vi "Save File Product Header Specific.vi"(8 "Error In":errorcluster, 10 "LV Program":T7=enum."DOE Stand", 11 "Appliance Details":T1 {"Dryer"."Dryer Initial IMC Data"."Maximum Weight (lbf)" format="%03_6g"; "Dryer"."Dryer Initial IMC Data"."Average Weight (lbf)" format="%03_6g"; "Dryer"."Dryer Initial IMC Data"."Minimum Weight (lbf)" format="%03_6g"; "Dryer"."Dryer Initial IMC Data"."CEF (lbf/kWh)" format="%03_6g"; "Dryer"."Dryer Initial IMC Data"."Actual Final RMC (%)" format="%03_6g"; "Dryer"."Dryer Initial IMC Data"."Tolerance(%)" format="%0#_6g"; "Dryer"."Dryer Initial IMC Data"."Bone Dry Wt(lbs)" format="%03_6g"; "Dryer"."Dryer Initial IMC Data"."RMC (Desired %)" format="%0#_6g"; "Dryer"."Dryer Initial IMC Data"."Actual Initial RMC (%)" format="%03_6g"; "Dryer"."Dryer Initial IMC Data"."Measured IMC (lbs)" format="%0#_6g"}) -> (0 "Error Out":errorcluster, 3 "array":string[][](array[string]))   [LabVIEW 2018, in "File Setup.lvlib"]
uses:
  File Setup.lvlib
  File Setup (Public)/Type Definition/Save File DOE LabView Program.ctl
  File Setup (Public)/Type Definition/Save File DISH Dishwasher Details.ctl
  <vilib>/Platform/fileVersionInfo.llb/FileVersionInformation.ctl
  Washer DOE/Type Definitions/DOE Appliance Common.ctl
  Custom Pallet Controls/Custom Pallet String.ctl
  File Setup (Public)/Type Definition/DPT IMC Data.ctl
  Washer DOE/Type Definitions/DOE Dryer Standard.ctl
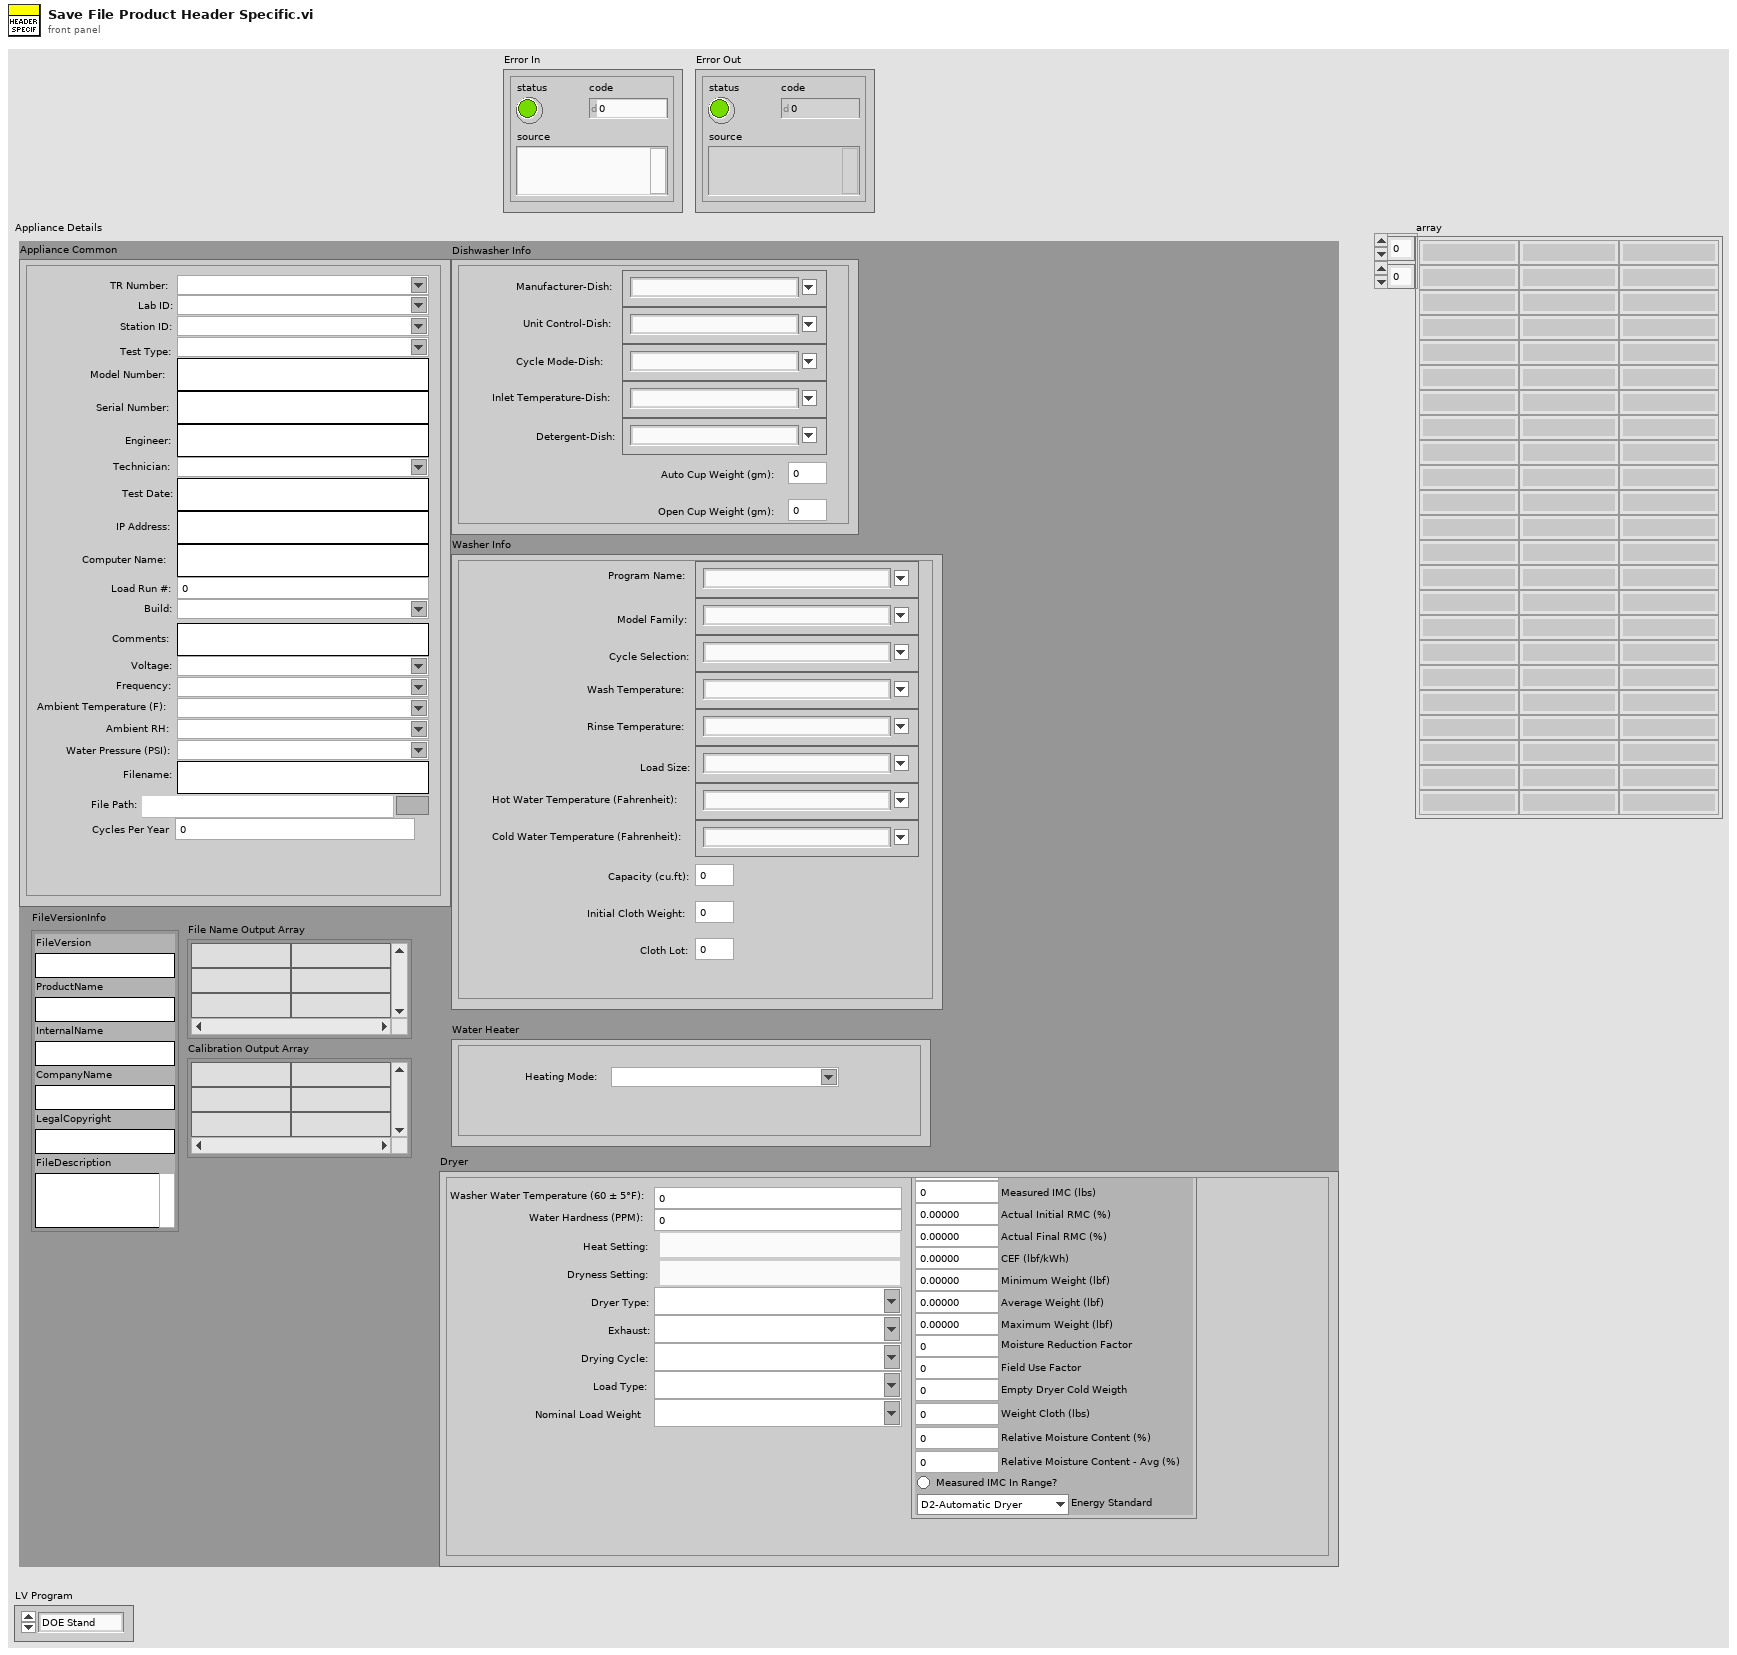
[diagram p1: front panel]
types:
  T1 = typedef "File Setup.lvlib/Save File DISH Dishwasher Details.ctl" = cluster{"FileVersionInfo":T2, "Dishwasher Info":cluster{"Open Cup Weight (gm):":dbl, "Auto Cup Weight (gm):":dbl, "Detergent-Dish:":string, "Inlet Temperature-Dish:":string, "Cycle Mode-Dish:":string, "Unit Control-Dish:":string, "Manufacturer-Dish:":string}, "Washer Info":cluster{"Hot Water Temperature (Fahrenheit):":string, "Cold Water Temperature (Fahrenheit):":string, "Capacity (cu.ft):":dbl, "Initial Cloth Weight:":dbl, "Cloth Lot:":i32, "Model Family:":string, "Program Name:":string, "Cycle Selection:":string, "Wash Temperature:":string, "Rinse Temperature:":string, "Load Size:":string}, "File Name Output Array":string[][], "Calibration Output Array":string[][], "Appliance Common":T3, "Water Heater":cluster{"Heating Mode:":string}, "Dryer":cluster{"Heat Setting:":T4, "Washer Water Temperature (60 ± 5°F):":u16, "Water Hardness (PPM):":u16, "Dryness Setting:":T4, "Dryer Type:":string, "Exhaust:":string, "Drying Cycle:":string, "Load Type:":string, "Nominal Load Weight":string, "Dryer Initial IMC Data":T5}}
  T2 = typedef "FileVersionInformation.ctl" = cluster{"FileVersion":string, "ProductName":string, "InternalName":string, "CompanyName":string, "LegalCopyright":string, "FileDescription":string}
  T3 = typedef "DOE Appliance Common.ctl" = cluster{"Engineer:":string, "Model Number:":string, "Serial Number:":string, "Comments:":string, "Station ID:":string, "Technician:":string, "TR Number:":string, "Lab ID:":string, "Voltage:":string, "Water Pressure (PSI):":string, "Test Date:":string, "Computer Name:":string, "IP Address:":string, "Ambient RH:":string, "Frequency:":string, "Build:":string, "Filename:":string, "Test Type:":string, "Load Run #:":i32, "Ambient Temperature (F):":string, "File Path:":path, "Cycles Per Year":u32}
  T4 = typedef "Custom Pallet String.ctl" = string
  T5 = typedef "DPT IMC Data.ctl" = cluster{"Measured IMC (lbs)":dbl, "Actual Initial RMC (%)":dbl, "RMC (Desired %)":dbl, "Bone Dry Wt(lbs)":dbl, "Tolerance(%)":dbl, "Actual Final RMC (%)":dbl, "CEF (lbf/kWh)":dbl, "Minimum Weight (lbf)":dbl, "Average Weight (lbf)":dbl, "Maximum Weight (lbf)":dbl, "Measured IMC In Range?":bool, "Moisture Reduction Factor":dbl, "Field Use Factor":dbl, "Empty Dryer Cold Weigth":dbl, "Energy Standard":T6, "Weight Cloth (lbs)":dbl, "Relative Moisture Content (%)":dbl, "Relative Moisture Content - Avg (%)":dbl}
  T6 = typedef "DOE Dryer Standard.ctl" = enum16{"D2-Automatic Dryer", "D2-Timer Dryer", "D1-Automatic Dryer", "D1-Timer Dryer", "Other"}
  T7 = typedef "File Setup.lvlib/Save File DOE LabView Program.ctl" = enum16{"No Name Found", "DOE Stand", "Dishwasher Kitchen", "Portable Stand", "HEWH", "Dryer", "Dryer WILT", "HCC", "PRAT", "HEWH RLT", "Refrigeration"}
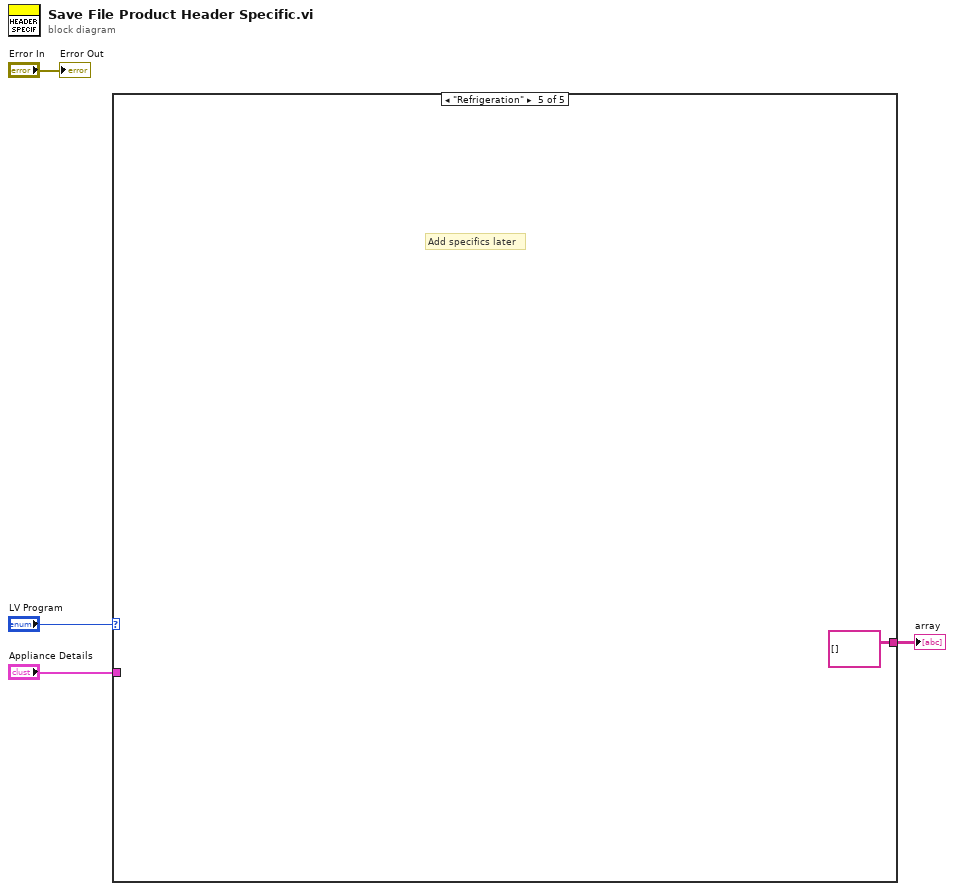
[diagram p0: block diagram]
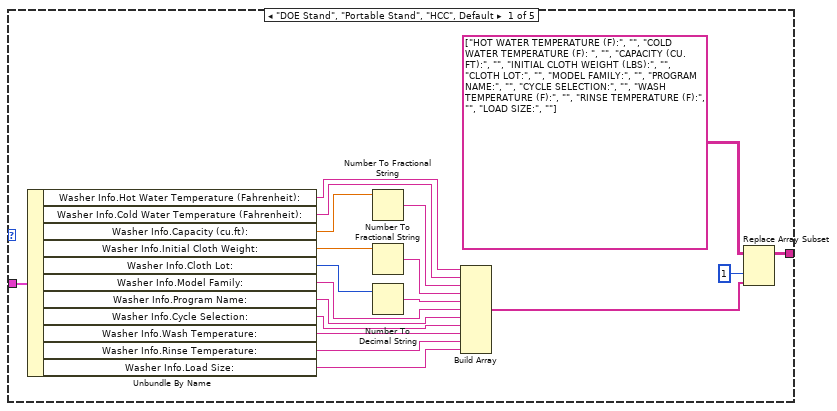
[diagram p2: hidden frame]
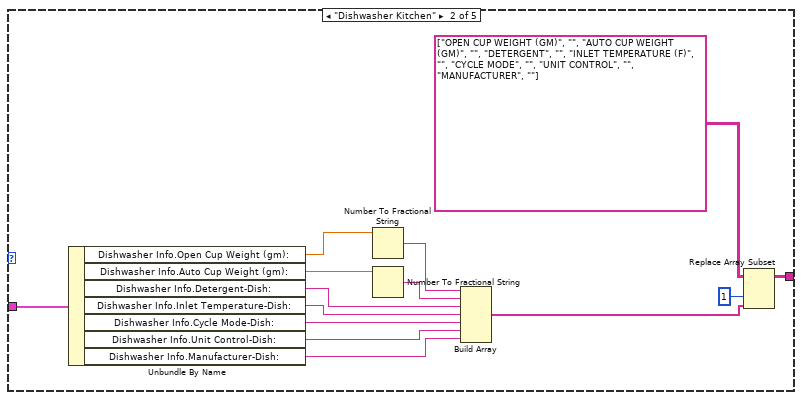
[diagram p3: hidden frame]
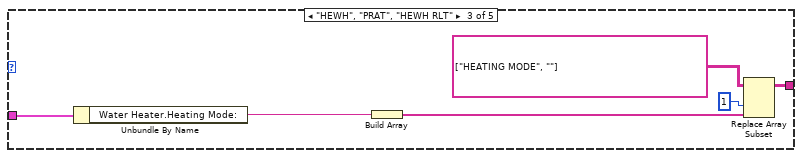
[diagram p4: hidden frame]
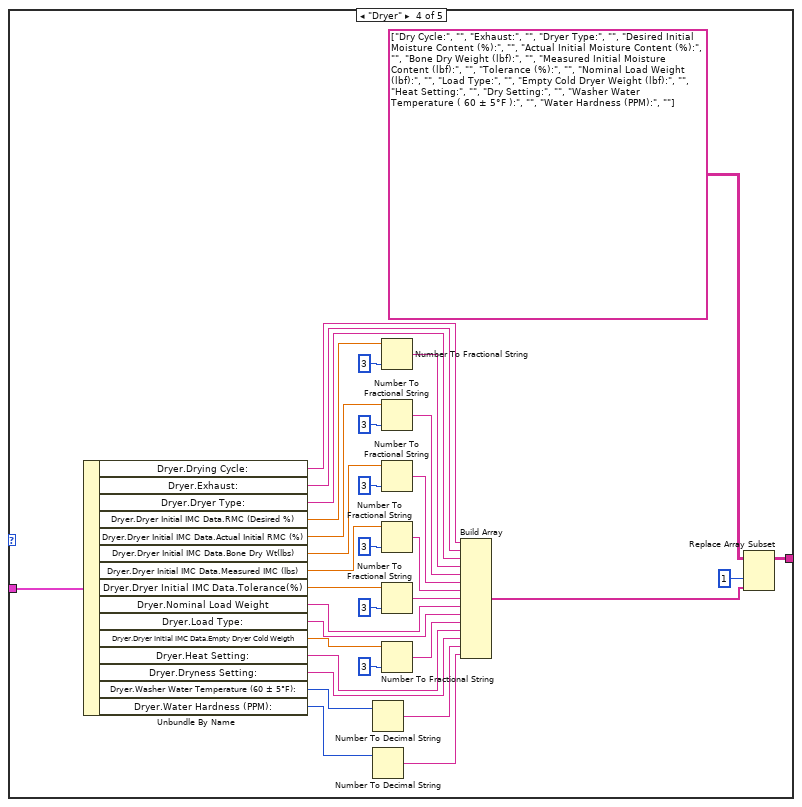
[diagram p5: hidden frame]
diagram:
  n1 = case shown="\"Refrigeration\"" "LV Program" {
    tunnel: "Appliance Details" -> [w23 w37 w39 w77 _]
    tunnel: [w5 w24 w38 w52 string[][] [] ("array")] -> w4
    frame "DOE Stand", "Portable Stand", "HCC", Default {
      n2 = Unbundle By Name(w23) -> ("Washer Info.Hot Water Temperature (Fahrenheit):"=w22:string, "Washer Info.Cold Water Temperature (Fahrenheit):"=w21:string, "Washer Info.Capacity (cu.ft):"=w20:dbl, "Washer Info.Initial Cloth Weight:"=w19:dbl, "Washer Info.Cloth Lot:"=w16:i32, "Washer Info.Model Family:"=w14:string, "Washer Info.Program Name:"=w13:string, "Washer Info.Cycle Selection:"=w12:string, "Washer Info.Wash Temperature:"=w11:string, "Washer Info.Rinse Temperature:"=w10:string, "Washer Info.Load Size:"=w9:string)
      n3 = Number To Fractional String(number=w20) -> (F-format string=w18:string)  [unwired: 3 in]
      n4 = Number To Fractional String(number=w19) -> (F-format string=w17:string)  [unwired: 3 in]
      n5 = Number To Decimal String(number=w16) -> (decimal integer string=w15:string)  [unwired: 1 in]
      n6 = Build Array(w22, w21, w18, w17, w15, w14, w13, w12, w11, w10, w9) -> (w7:string[])
      n7 = Replace Array Subset(array=string[][] [["HOT WATER TEMPERATURE (F):", ""], ["COLD WATER TEMPERATURE (F): ", ""], ["CAPACITY (CU.FT):", ""], ["INITIAL CLOTH WEIGHT (LBS):", ""], ["CLOTH LOT:", ""], ["MODEL FAMILY:", ""], ["PROGRAM NAME:", ""], ["CYCLE SELECTION:", ""], ["WASH TEMPERATURE (F):", ""], ["RINSE TEMPERATURE (F):", ""], ["LOAD SIZE:", ""]], new element=w7, index (col)=1 ("disabled index (col)")) -> (w5:string[][])  [unwired: 1 in]
    }
    frame "Dishwasher Kitchen" {
      n8 = Unbundle By Name(w37) -> ("Dishwasher Info.Open Cup Weight (gm):"=w36:dbl, "Dishwasher Info.Auto Cup Weight (gm):"=w35:dbl, "Dishwasher Info.Detergent-Dish:"=w32:string, "Dishwasher Info.Inlet Temperature-Dish:"=w31:string, "Dishwasher Info.Cycle Mode-Dish:"=w30:string, "Dishwasher Info.Unit Control-Dish:"=w29:string, "Dishwasher Info.Manufacturer-Dish:"=w28:string)
      n9 = Number To Fractional String(number=w36) -> (F-format string=w34:string)  [unwired: 3 in]
      n10 = Number To Fractional String(number=w35) -> (F-format string=w33:string)  [unwired: 3 in]
      n11 = Build Array(w34, w33, w32, w31, w30, w29, w28) -> (w27:string[])
      n12 = Replace Array Subset(array=string[][] [["OPEN CUP WEIGHT (GM)", ""], ["AUTO CUP WEIGHT (GM)", ""], ["DETERGENT", ""], ["INLET TEMPERATURE (F)", ""], ["CYCLE MODE", ""], ["UNIT CONTROL", ""], ["MANUFACTURER", ""]], new element=w27, index (col)=1 ("disabled index (col)")) -> (w24:string[][])  [unwired: 1 in]
    }
    frame "HEWH", "PRAT", "HEWH RLT" {
      n13 = Unbundle By Name(w39) -> ("Water Heater.Heating Mode:"=w43:string)
      n14 = Build Array(w43) -> (w42:string[])
      n15 = Replace Array Subset(array=string[][] [["HEATING MODE", ""]], new element=w42, index (col)=1 ("disabled index (col)")) -> (w38:string[][])  [unwired: 1 in]
    }
    frame "Dryer" {
      n16 = Unbundle By Name(w77) -> ("Dryer.Drying Cycle:"=w74:string, "Dryer.Exhaust:"=w73:string, "Dryer.Dryer Type:"=w72:string, "Dryer.Dryer Initial IMC Data.RMC (Desired %)"=w71:dbl, "Dryer.Dryer Initial IMC Data.Actual Initial RMC (%)"=w69:dbl, "Dryer.Dryer Initial IMC Data.Bone Dry Wt(lbs)"=w67:dbl, "Dryer.Dryer Initial IMC Data.Measured IMC (lbs)"=w65:dbl, "Dryer.Dryer Initial IMC Data.Tolerance(%)"=w63:dbl, "Dryer.Nominal Load Weight"=w61:string, "Dryer.Load Type:"=w60:string, "Dryer.Dryer Initial IMC Data.Empty Dryer Cold Weigth"=w51:dbl, "Dryer.Heat Setting:"=w59:T4, "Dryer.Dryness Setting:"=w58:T4, "Dryer.Washer Water Temperature (60 ± 5°F):"=w57:u16, "Dryer.Water Hardness (PPM):"=w55:u16)
      n17 = Number To Decimal String(number=w57) -> (decimal integer string=w56:string)  [unwired: 1 in]
      n18 = Number To Decimal String(number=w55) -> (decimal integer string=w54:string)  [unwired: 1 in]
      n19 = Number To Fractional String(number=w71, precision (6)=i16 3) -> (F-format string=w70:string)  [unwired: 2 in]
      n20 = Number To Fractional String(number=w69, precision (6)=i16 3) -> (F-format string=w68:string)  [unwired: 2 in]
      n21 = Number To Fractional String(number=w67, precision (6)=i16 3) -> (F-format string=w66:string)  [unwired: 2 in]
      n22 = Number To Fractional String(number=w65, precision (6)=i16 3) -> (F-format string=w64:string)  [unwired: 2 in]
      n23 = Number To Fractional String(number=w63, precision (6)=i16 3) -> (F-format string=w62:string)  [unwired: 2 in]
      n24 = Number To Fractional String(number=w51, precision (6)=i16 3) -> (F-format string=w50:string)  [unwired: 2 in]
      n25 = Build Array(w74, w73, w72, w70, w68, w66, w64, w62, w61, w60, w50, w59, w58, w56, w54) -> (w53:T4[])
      n26 = Replace Array Subset(array=string[][] [["Dry Cycle:", ""], ["Exhaust:", ""], ["Dryer Type:", ""], ["Desired Initial Moisture Content (%):", ""], ["Actual Initial Moisture Content (%):", ""], ["Bone Dry Weight (lbf):", ""], ["Measured Initial Moisture Content (lbf):", ""], ["Tolerance (%):", ""], ["Nominal Load Weight (lbf):", ""], ["Load Type:", ""], ["Empty Cold Dryer Weight (lbf):", ""], ["Heat Setting:", ""], ["Dry Setting:", ""], ["Washer Water Temperature ( 60 ± 5°F ):", ""], ["Water Hardness (PPM):", ""]], new element=w53, index (col)=1 ("disabled index (col)")) -> (w52:string[][])  [unwired: 1 in]
    }
    frame "Refrigeration" {
      # "Add specifics later"
    }
  }
  "array" <- w4
  "Error Out" <- "Error In"
